vi "flow_chart.vi"() -> ()   [LabVIEW 2015]
panel:
  in  "Command 2":string
  out "?":sgl(graph)
  out "?":sgl(graph)
  out "?":sgl(graph)
  in  "?":bool
  in  "?":bool
  in  "?":bool
  in  "Command 3":string
  out "flow 3":sgl caption="flow" format="%.3g"
  out "flow 2":sgl caption="flow" format="%.3g"
  out "flow":sgl format="%.3g"
  in  "Command":string
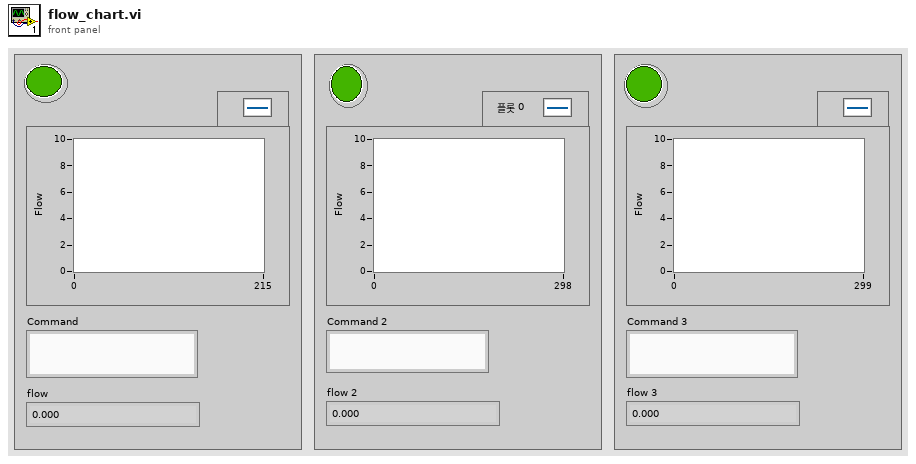
[diagram p1: front panel]
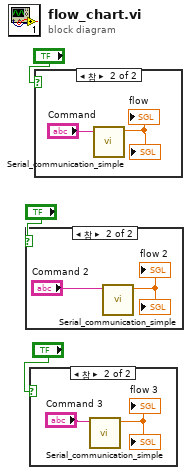
[diagram p0: block diagram]
diagram:
  n1 = case shown="참" "?" {
    frame False {
    }
    frame True {
      n2 = call "Serial_communication_simple.vi"("Command"="Command 2") -> ("flow"=→"?" →"flow 2":sgl)  [unwired: 10 in]
    }
  }
  n3 = case shown="참" "?" {
    frame False {
    }
    frame True {
      n4 = call "Serial_communication_simple.vi"("Command"="Command 3") -> ("flow"=→"?" →"flow 3":sgl)  [unwired: 10 in]
    }
  }
  n5 = case shown="참" "?" {
    frame False {
    }
    frame True {
      n6 = call "Serial_communication_simple.vi"("Command"="Command") -> ("flow"=→"?" →"flow":sgl)  [unwired: 10 in]
    }
  }
